vi "Assert Less Or Equal_Variant.vi"(4 "Execution time (s)":dbl=-1.0, 6 "error code (1)":i32=1, 7 "Label":string, 8 "error in":errorcluster, 10 "Y":variant, 11 "X":variant) -> (0 "error out":errorcluster, 2 "Properties":refnum<class "Properties.Assert.lvclass">)   [LabVIEW 2021, in "Bananas.lvlib"]
uses:
  Bananas.lvlib
  <vilib>/addons/_JKI Toolkits/Caraya/classes/Properties.Assert/Properties.Assert.lvclass
  Banana/Banana.lvclass/Banana.ctl
  AssertTrue/AssertTrue.lvclass
  C:/Repositories/LVOS/Bananas/lv-src/Bananas/BananaPeel/BananaPeel.lvclass
  <vilib>/addons/_JKI Toolkits/Caraya/classes/Assert/Assert.lvclass
  Banana/Banana.lvclass
  AssertCompareValue/AssertCompareValue.lvclass
  C:/Repositories/LVOS/Bananas/lv-src/Bananas/AssertCompareValue/AssertCompareValue.lvclass
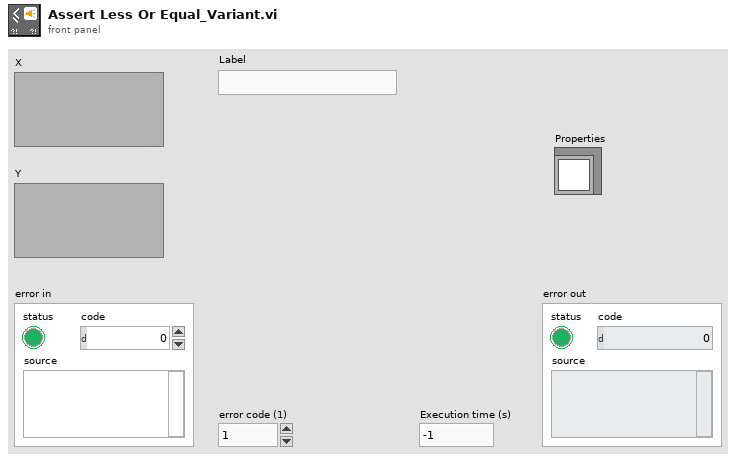
[diagram p1: front panel]
types:
  T1 = typedef "Bananas.lvlib/Assertion Strategies -- cluster.ctl" = cluster{"AssertTrue":refnum<class "AssertTrue.lvclass">, "AssertFalse":refnum<class "AssertFalse.lvclass">, "AssertEqualValue":refnum<class "AssertEqualValue.lvclass">, "AssertEqualType":refnum<class "AssertEqualType.lvclass">, "AssertCompareValue":refnum<class "AssertCompareValue.lvclass">}
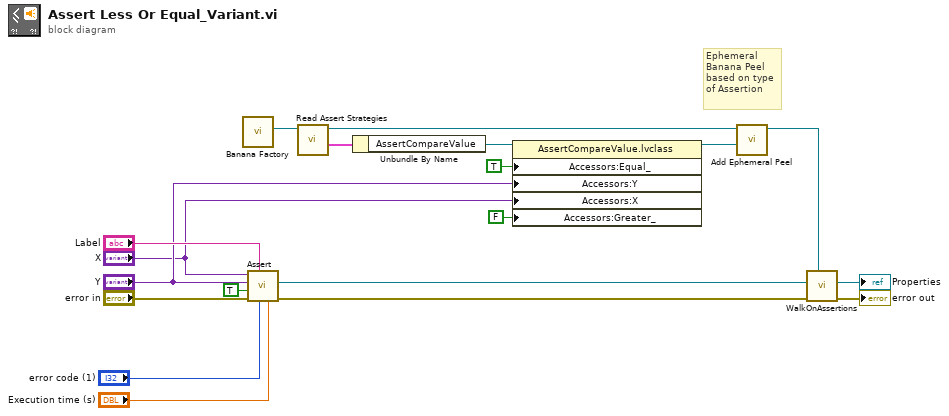
[diagram p0: block diagram]
diagram:
  # "Ephemeral\nBanana Peel\nbased on type\nof Assertion"
  n1 = call "Banana Factory.vi"() -> ("Bunch"=w9:refnum<class "Banana.lvclass">)  [unwired: 10 in, 1 out]
  n2 = call-poly <vilib>:"Assert.vi"("Execution time (s)"="Execution time (s)", "error code (1)"="error code (1)", "Label"="Label", "error in (no error)"="error in", "Register with caller test (F)"=TRUE, "Y"="Y", "X"="X") -> ("error out"=w14:errorcluster, "Properties.Assert"=w12:refnum<class "Properties.Assert.lvclass">)  [unwired: 3 in]
  n3 = call "Read Assert Strategies.vi"("Banana in"=w9) -> ("Strategies"=w4:T1, "Banana out"=w8:refnum<class "Banana.lvclass">)  [unwired: 9 in]
  n4 = Unbundle By Name(w4) -> ("AssertCompareValue"=w7:refnum<class "AssertCompareValue.lvclass">)
  n5 = property class="AssertCompareValue.lvclass"(reference=w7, "Accessors:Equal_"=TRUE ("Equal_"), "Accessors:Y"="Y", "Accessors:X"="X", "Accessors:Greater_"=FALSE ("Greater_")) -> (reference out=w3:refnum<class "AssertCompareValue.lvclass">)  [unwired: 1 in, 1 out]
  n6 = call "Add Ephemeral Peel.vi"("BananaPeel"=w3, "Bunch"=w8) -> ("Bunch"=w10:refnum<class "Banana.lvclass">)  [unwired: 9 in]
  n7 = call "WalkOnAssertions.vi"("Bunch"=w10, "error in (no error)"=w14, "Properties"=w12) -> ("error out"=→"error out":errorcluster, "Properties out"=→"Properties":refnum<class "Properties.Assert.lvclass">)  [unwired: 7 in]
